vi "Log Data.vi"(8 "error in (no error)":errorcluster, 10 "tdms file":refnum<k34>, 11 "Acquired Result in":refnum<class "Acquired Result.lvclass">) -> (0 "error out":errorcluster, 2 "tdms file out":refnum<k34>, 3 "Acquired Result out":refnum<class "Acquired Result.lvclass">)   [LabVIEW 2016, in "Acquired Result.lvclass"]
uses:
  Acquired Result.lvclass
  Acquired Result.lvclass/Acquired Result.ctl
  Read Group.vi
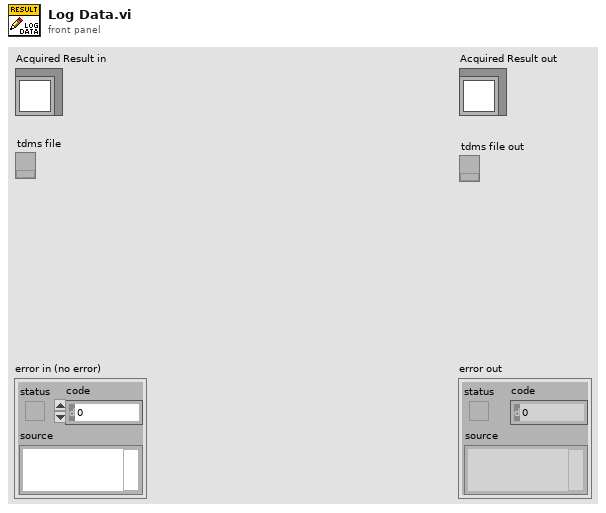
[diagram p1: front panel]
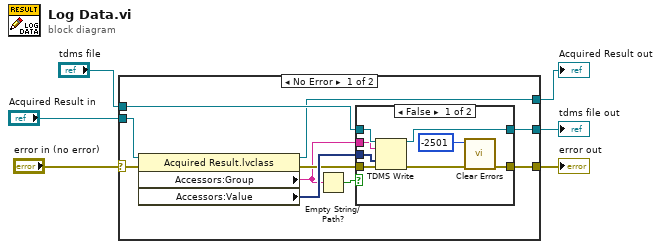
[diagram p0: block diagram]
diagram:
  n1 = case shown="No Error" "error in (no error)" {
    selector: "error in (no error)" -> [w10 w27]
    tunnel: "Acquired Result in" -> [w16 w29]
    tunnel: "tdms file" -> [w15 w28]
    tunnel: [w14 w28] -> w4
    tunnel: [w13 w29] -> w3
    tunnel: [w9 w27] -> w2
    frame No Error {
      n2 = property class="Acquired Result.lvclass"(reference=w16, error in=w10) -> (reference out=w13:refnum<class "Acquired Result.lvclass">, error out=w11:errorcluster, "Accessors:Group"=w7:string, "Accessors:Value"=w12:dynamicdata)
      n3 = Empty String/Path?(string/path=w7) -> (empty?=w8:bool)
      n4 = case shown="False" w8 {
        tunnel: w15 -> [w24 w26]
        tunnel: [w23 w26] -> w14
        tunnel: w7 -> [w22 _]
        tunnel: w12 -> [w21 _]
        tunnel: w11 -> [w19 w25]
        tunnel: [w18 w25] -> w9
        frame False {
          n5 = TDMS Write(0:w24, 5:w22, 9:w21, 11:w19) -> (4:w23:refnum<k34>, 15:w20:errorcluster)  [unwired: 2 in, 2 out]
          n6 = call <vilib>:"Clear Errors.vi"("error in (no error)"=w20, "specific error code to clear (0: all)"=-2501) -> ("error out"=w18:errorcluster)  [unwired: 4 in, 1 out]
        }
        frame True {
        }
      }
    }
    frame Error {
    }
  }
  "error out" <- w2
  "Acquired Result out" <- w3
  "tdms file out" <- w4
